vi "Configuration-ReadString.vi"(7 "error in (no error)":errorcluster caption="错误输入（无错误）", 8 "default value":string caption="默认值", 9 "key":string caption="键", 10 "section":string caption="段") -> (0 "error out":errorcluster caption="错误输出", 2 "value":string caption="值", 3 "found?":bool caption="已找到？")   [LabVIEW 2014]
uses:
  <vilib>/Utility/config.llb/Read Key (String).vi
  <vilib>/Utility/config.llb/NI_LVConfig.lvlib
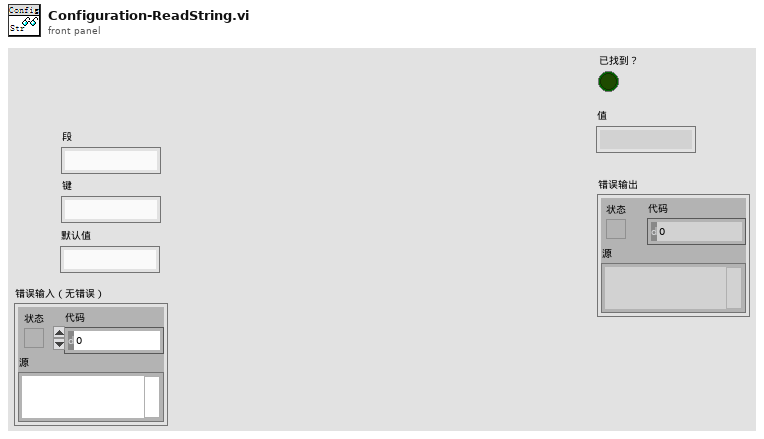
[diagram p1: front panel]
types:
  T1 = typedef "NI_LVConfig.lvlib/Config Data RefNum.ctl" = refnum<k1>
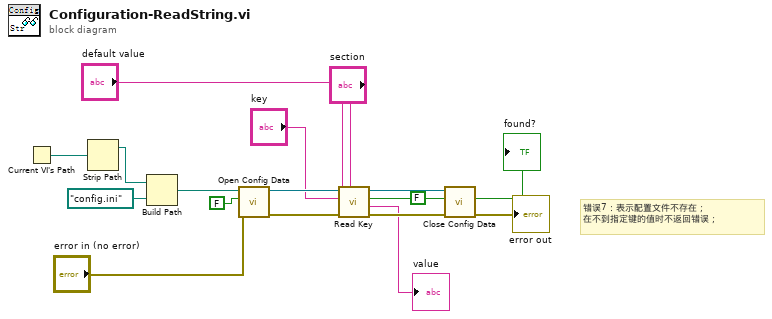
[diagram p0: block diagram]
diagram:
  # "错误7：表示配置文件不存在；\n在不到指定键的值时不返回错误；"
  n1 = Current VI's Path() -> (path=w3:path)
  n2 = Strip Path(path=w3) -> (stripped path=w2:path)  [unwired: 1 out]
  n3 = Build Path(base path=w2, name or relative path=path "config.ini" ("default name")) -> (appended path=w12:path)
  n4 = call <vilib>:"Open Config Data.vi"("error in (no error)"="error in (no error)", "create file if necessary (T)"=FALSE ("create file if necessary? (T)"), "configuration file path"=w12) -> ("error out"=w17:errorcluster, "refnum"=w16:T1)  [unwired: 6 in, 1 out]
  n5 = call-poly <vilib>:"Read Key.vi"("section"="section", "error in (no error)"=w17, "default value"="default value", "key"="key", "refnum"=w16) -> ("error out"=w11:errorcluster, "value"=→"value":string, "found?"=→"found?":bool, "refnum out"=w10:T1)  [unwired: 1 in, 2 out]
  n6 = call <vilib>:"Close Config Data.vi"("error in (no error)"=w11, "write file if changed (T)"=FALSE ("write configuration file? (T)"), "refnum"=w10) -> ("error out"=→"error out":errorcluster)  [unwired: 8 out]
